vi "配置读取.vi"(8 "error in (no error)":errorcluster caption="错误输入（无错误）") -> (0 "error out":errorcluster caption="错误输出")   [LabVIEW 2016, in "斯坦道总氮.lvlib"]
uses:
  <vilib>/Utility/config.llb/NI_LVConfig.lvlib
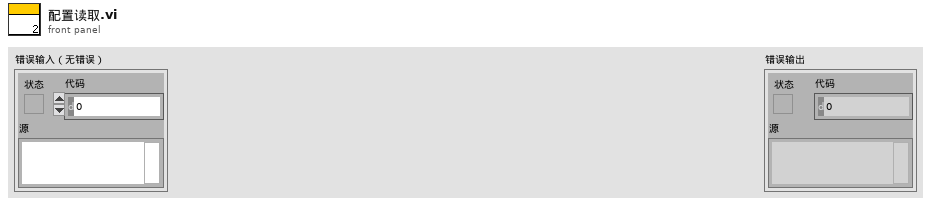
[diagram p1: front panel]
types:
  T1 = typedef "NI_LVConfig.lvlib/Config Data RefNum.ctl" = refnum<k1>
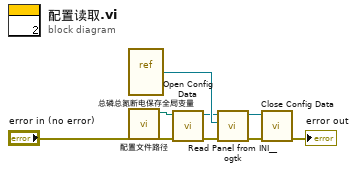
[diagram p0: block diagram]
diagram:
  n1 = vi-ref "总磷总氮断电保存全局变量.vi"() -> (w5:refnum<vi>)
  n2 = call "配置文件路径.vi"() -> ("appended path"=w1:path)  [unwired: 11 in]
  n3 = call <vilib>:"Open Config Data.vi"("error in (no error)"="error in (no error)", "configuration file path"=w1) -> ("error out"=w7:errorcluster, "refnum"=w4:T1)  [unwired: 7 in, 1 out]
  n4 = call <userlib>:"Read Panel from INI__ogtk.vi"("error in (no error)"=w7, "VI ref"=w5, "refnum"=w4) -> ("error out"=w8:errorcluster, "refnum out"=w6:T1)  [unwired: 7 in]
  n5 = call <vilib>:"Close Config Data.vi"("error in (no error)"=w8, "refnum"=w6) -> ("error out"=→"error out":errorcluster)  [unwired: 8 in, 1 out]
